vi "Process Objects1.vi"(9 "read device ID code":T1(ring), 10 "object ID":u8, 11 "objects":cluster{"object ID":u8, "value":string}[](array[cluster]) {"object ID" format="%x"}) -> (0 "object data":u8[](array[numeric]), 1 "object count":u8, 2 "next object ID":u8, 3 "more follows":u8)   [LabVIEW 2021, in "NI_modbus_upd.lvlib" / "Standard Data Model1.lvclass"]
doc: "This VI accepts the objects of the device and the requested object information and generates the required object data and metadata."
uses:
  Standard Data Model1.lvclass
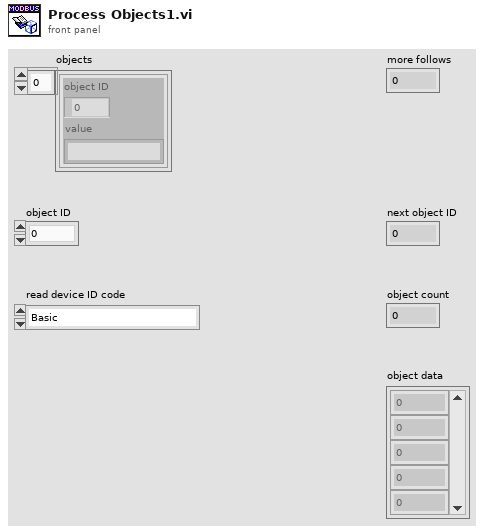
[diagram p1: front panel]
types:
  T1 = enum8{"Basic", "Regular", "Extended", "Specific"}
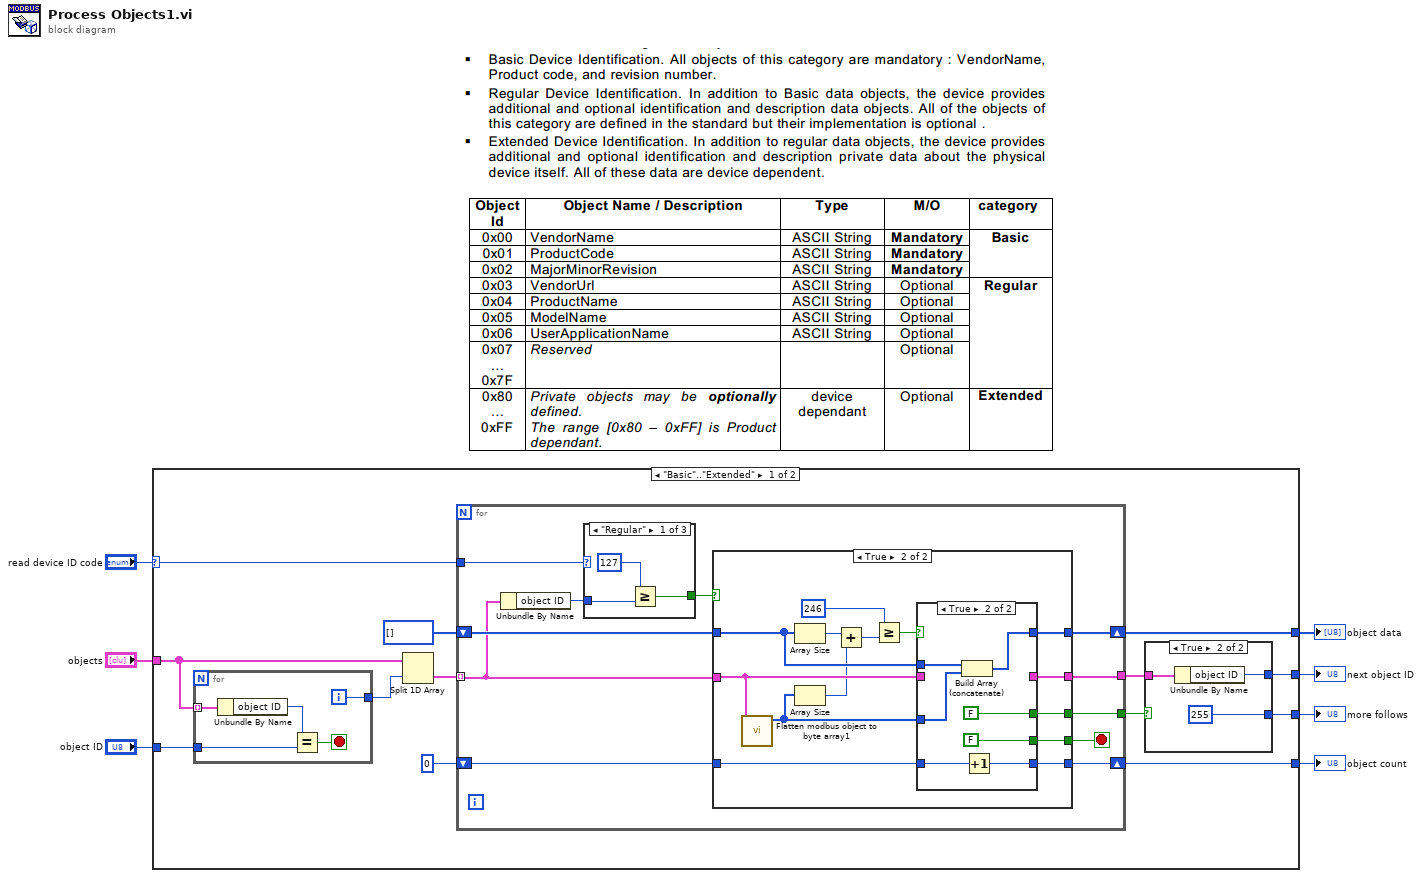
[diagram p0: block diagram]
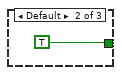
[diagram p2: hidden frame]
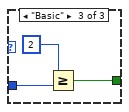
[diagram p3: hidden frame]
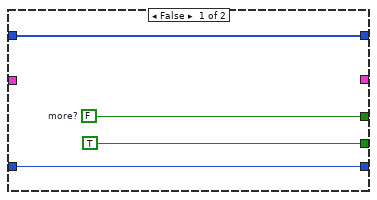
[diagram p4: hidden frame]
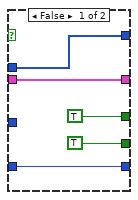
[diagram p5: hidden frame]
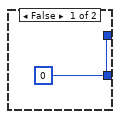
[diagram p6: hidden frame]
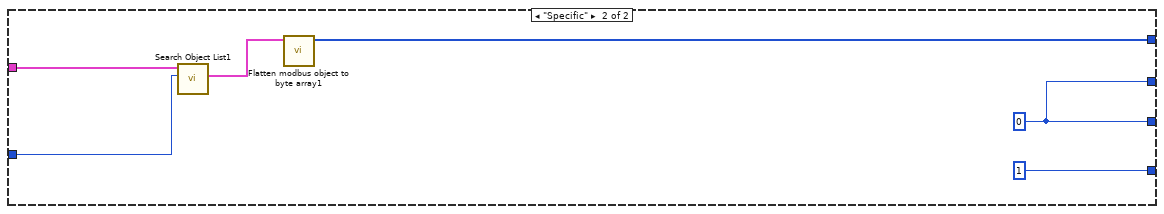
[diagram p7: hidden frame]
diagram:
  n1 = case shown="\"Basic\"..\"Extended\"" "read device ID code" {
    selector: "read device ID code" -> [w10 _]
    tunnel: "objects" -> [w19 w83]
    tunnel: [w13 u8 1] -> w5
    tunnel: [w16 w80] -> w4
    tunnel: [w15 w80] -> w3
    tunnel: "object ID" -> [w20 w79]
    tunnel: [w11 w78] -> w1
    frame "Basic".."Extended" {
      n2 = for {
        tunnel: w19 -> [w77] mode=indexing
        tunnel: w20 -> [w76]
        tunnel: [w73] -> w18
        i -> [w73]
        stop <- w74 stop-if-true
        n3 = Unbundle By Name(w77) -> ("object ID"=w75:u8)
        n4 = Equal?(x=w75, y=w76) -> (x = y?=w74:bool)
      }
      n5 = Split 1D Array(array=w19, index=w18) -> (second subarray=w17:cluster{"object ID":u8, "value":string}[])  [unwired: 1 out]
      n6 = for {
        shift-right: [w28] -> w13
        shift-left: 0 -> [w29]
        shift-right: [w30] -> w11
        shift-left: u8[] [] -> [w31]
        tunnel: w17 -> [w22] mode=indexing
        tunnel: w10 -> [w27]
        tunnel: [w24] -> w9
        tunnel: [w23] -> w8
        stop <- w21 stop-if-true
        n7 = Unbundle By Name(w22) -> ("object ID"=w26:u8)
        n8 = case shown="\"Regular\"" w27 {
          tunnel: w26 -> [w32 _ w36]
          tunnel: [w34 TRUE w38] -> w25
          frame "Regular" {
            n9 = Greater Or Equal?(x=u8 127 ("y"), y=w32) -> (x >= y?=w34:bool)
          }
          frame Default {
          }
          frame "Basic" {
            n10 = Greater Or Equal?(x=u8 2 ("y"), y=w36) -> (x >= y?=w38:bool)
          }
        }
        n11 = case shown="True" w25 {
          tunnel: w31 -> [w41 w54]
          tunnel: [w41 w53] -> w30
          tunnel: w29 -> [w40 w52]
          tunnel: [w40 w51] -> w28
          tunnel: [TRUE w50] -> w21
          tunnel: w22 -> [_ w49]
          tunnel: [w39 w47] -> w24
          tunnel: [_ w48] -> w23
          frame False {
            w39 = FALSE  # more?
          }
          frame True {
            n12 = call "Flatten modbus object to byte array1.vi"("object"=w49) -> ("byte array"=w55:u8[])  [unwired: 10 in]
            n13 = Array Size(array=w54) -> (size(s)=w46:i32)
            n14 = Array Size(array=w55) -> (size(s)=w45:i32)
            n15 = Add(x=w46, y=w45) -> (x+y=w44:i32)
            n16 = Greater Or Equal?(x=246 ("y"), y=w44) -> (x >= y?=w56:bool)
            n17 = case shown="True" w56 {
              tunnel: w55 -> [_ w66]
              tunnel: w54 -> [w60 w68]
              tunnel: [w60 w67] -> w53
              tunnel: w52 -> [w61 w65]
              tunnel: [w61 w64] -> w51
              tunnel: [TRUE FALSE] -> w50
              tunnel: w49 -> [w58 _]
              tunnel: [w58 _] -> w48
              tunnel: [TRUE FALSE] -> w47
              frame False {
              }
              frame True {
                n18 = Build Array (concatenate)(w68, w66) -> (w67:u8[])
                n19 = Increment(x=w65) -> (x+1=w64:i32)
              }
            }
          }
        }
      }
      n20 = case shown="True" w9 {
        tunnel: [w69 u8 255] -> w16
        tunnel: [w69 w70] -> w15
        tunnel: w8 -> [_ w71]
        frame False {
          w69 = u8 0
        }
        frame True {
          n21 = Unbundle By Name(w71) -> ("object ID"=w70:u8)
        }
      }
    }
    frame "Specific" {
      w80 = u8 0
      n22 = call "Search Object List1.vi"("object ID"=w79, "objects"=w83) -> ("object"=w82:cluster{"object ID":u8, "value":string})  [unwired: 7 in, 2 out]
      n23 = call "Flatten modbus object to byte array1.vi"("object"=w82) -> ("byte array"=w78:u8[])  [unwired: 10 in]
    }
  }
  "object data" <- w1
  "next object ID" <- w3
  "more follows" <- w4
  "object count" <- w5
